vi "Ribbon Control.vi"() -> ()   [LabVIEW 2014]
panel:
  in  "1":bool
  in  "0":bool
  out "Tab Control":enum32{"0", "1"}(tab)
  in  "Tab 1 Group 2":enum32{"Page 2"}(tab)
  in  "Button Rack Center 4":bool
  in  "Button Rack Center 3":bool
  in  "Button Rack Right 2":bool
  in  "Button Rack Left 2":bool
  in  "Button Rack Center 2":bool
  in  "Button Rack Right":bool
  in  "Button Rack Left":bool
  in  "Button Rack Center":bool
  in  "String":string
  out "Ring 2":u16(ring)
  in  "Tab 1 Group 1":enum32{"Page 2"}(tab)
  in  "Add Button":bool
  in  "Save Button":bool
  in  "New Button":bool
  out "Ring":u16(ring)
  in  "Tab 2 Group 1":enum32{"Page 2"}(tab)
  in  "Add Button 3":bool
  in  "Save Button 3":bool
  in  "New Button 3":bool
  in  "Add Button 2":bool
  in  "Save Button 2":bool
  in  "New Button 2":bool
  out "Ring 3":u16(ring)
  out "Waveform Graph":dynamicdata(graph)
  in  "Frequency":dbl(slide) scale=0.0..10.0 scale format="%#_6p"
  in  "Amplitude":dbl(slide) scale=0.0..10.0
  in  "stop":bool
  # "Tab 1"
  # "Group Title"
  # "Group Title"
  # "Tab 2"
  # "Group Title"
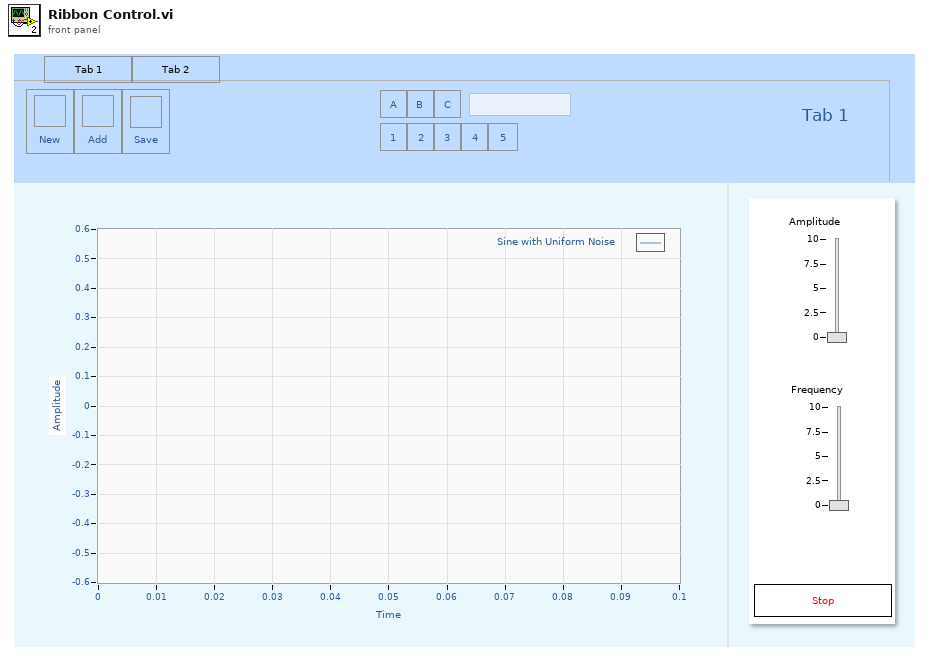
[diagram p1: front panel]
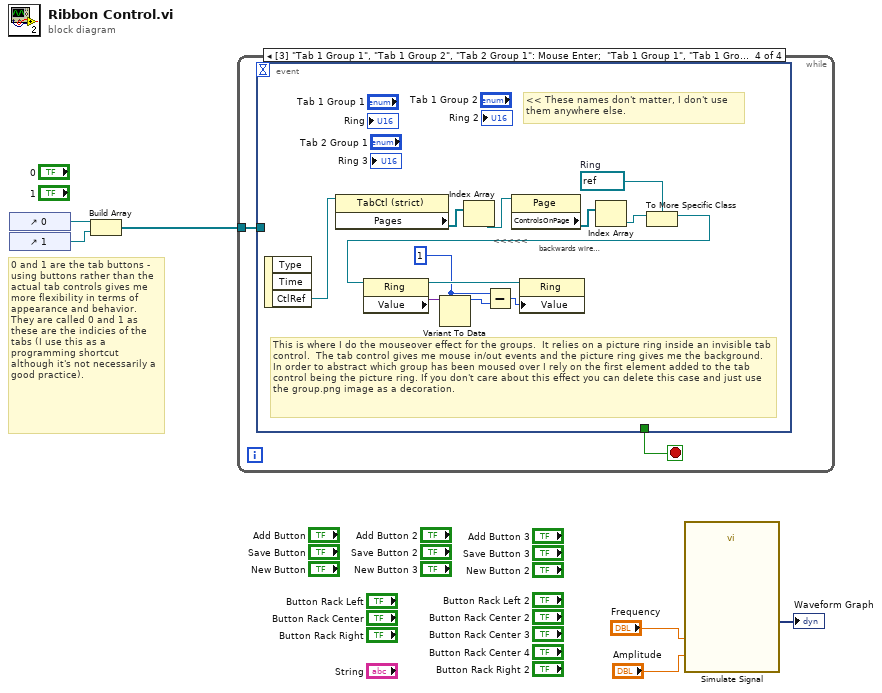
[diagram p0: block diagram]
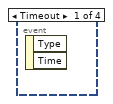
[diagram p2: hidden frame]
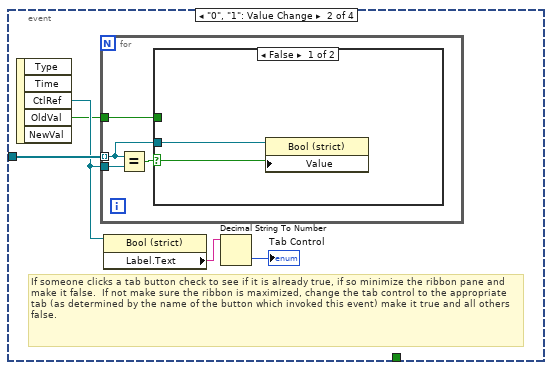
[diagram p3: hidden frame]
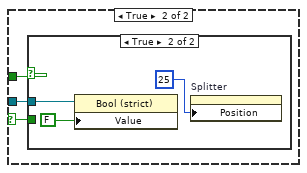
[diagram p4: hidden frame]
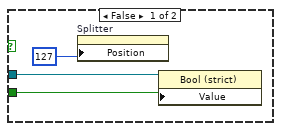
[diagram p5: hidden frame]
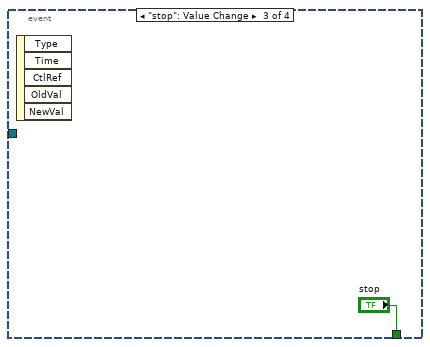
[diagram p6: hidden frame]
diagram:
  # "0 and 1 are the tab buttons - using buttons rather than the actual tab controls gives me more flexibility in terms of appearance and behavior.  They are called 0 and 1 as these are the indicies of the tabs (I use this as a programming shortcut although it's not necessarily a good practice)."
  n1 = control-ref of="0"() -> (w6:refnum<vi>)
  n2 = control-ref of="1"() -> (w5:refnum<vi>)
  n3 = Build Array(w6, w5) -> (w4:refnum<vi>[])
  n4 = while {
    tunnel: w4 -> [w8]
    stop <- w7 stop-if-true
    n5 = event shown="[3] \"Tab 1 Group 1\", \"Tab 1 Group 2\", \"Tab 2 Group 1\": Mouse Enter;  \"Tab 1 Group 1\", \"Tab 1 Group 2\", \"Tab 2 Group 1\": Mouse Leave" {
      selector: _ -> [_ _ _ _]
      dyn-events: _ -> [_ _ _ _]
      timeout: _ -> [_ _ _ _]
      tunnel: w8 -> [_ w11 _ _]
      tunnel: [_ _ "stop" _] -> w7
      event Timeout {
        n6 = event-data() -> ()  [unwired: 1 in, 2 out]
      }
      event "0", "1": Value Change {
        # "If someone clicks a tab button check to see if it is already true, if so minimize the ribbon pane and make it false.  If not make sure the ribbon is maximized, change the tab control to the appropriate tab (as determined by the name of the button which invoked this event) make it true and all others false."
        n7 = event-data() -> ("CtlRef"=w10:refnum<vi>, "OldVal"=w9:bool)  [unwired: 1 in, 3 out]
        n8 = for {
          tunnel: w11 -> [w16] mode=indexing
          tunnel: w10 -> [w17]
          tunnel: w9 -> [w14]
          n9 = Equal?(x=w16, y=w17) -> (x = y?=w15:bool)
          n10 = case shown="False" w15 {
            selector: w15 -> [w18 w22]
            tunnel: w16 -> [w19 w21]
            tunnel: w14 -> [_ w20]
            frame False {
              n11 = property on="Property Node" class="Bool (strict)"(reference=w19, "Value"=w18) -> ()  [unwired: 1 in, 2 out]
            }
            frame True {
              n12 = case shown="True" w20 {
                tunnel: w22 -> [w25 _]
                tunnel: w21 -> [w24 w27]
                frame False {
                  n13 = property on="Splitter" class="Splitter"("Position"=127 ("Splitter Position")) -> ()  [unwired: 2 in, 2 out]
                  n14 = property on="Property Node" class="Bool (strict)"(reference=w24, "Value"=w25) -> ()  [unwired: 1 in, 2 out]
                }
                frame True {
                  n15 = property on="Property Node" class="Bool (strict)"(reference=w27, "Value"=FALSE) -> ()  [unwired: 1 in, 2 out]
                  n16 = property on="Splitter" class="Splitter"("Position"=25 ("Splitter Position")) -> ()  [unwired: 2 in, 2 out]
                }
              }
            }
          }
        }
        n17 = property class="Bool (strict)"(reference=w10) -> ("Label.Text"=w13:string)  [unwired: 1 in, 2 out]
        n18 = Decimal String To Number(string=w13) -> (number=→"Tab Control":i32)  [unwired: 2 in, 1 out]
      }
      event "stop": Value Change {
        n19 = event-data() -> ()  [unwired: 1 in, 5 out]
      }
      event "Tab 1 Group 1", "Tab 1 Group 2", "Tab 2 Group 1": Mouse Enter; "Tab 1 Group 1", "Tab 1 Group 2", "Tab 2 Group 1": Mouse Leave {
        w31 = u16 1 ("Ring")
        w36 = refnum<vi> refnum  # Ring
        # "backwards wire (sorry!)"
        # "<< These names don't matter, I don't use\nthem anywhere else."
        # "This is where I do the mouseover effect for the groups.  It relies on a picture ring inside an invisible tab control.  The tab control gives me mouse in/out events and the picture ring gives me the background.  In order to abstract which group has been moused over I rely on the first element added to the tab control being the picture ring. If you don't care about this effect you can delete this case and just use the group.png image as a decoration."
        # "<<<<<"
        n20 = event-data() -> ("CtlRef"=w41:refnum<vi>)  [unwired: 1 in, 2 out]
        n21 = property class="TabCtl (strict)"(reference=w41) -> ("Pages"=w40:refnum<vi>[])  [unwired: 1 in, 2 out]
        n22 = Index Array(array=w40) -> (element=w39:refnum<vi>)  [unwired: 1 in]
        n23 = property class="Page"(reference=w39) -> ("ControlsOnPage"=w38:refnum<vi>[])  [unwired: 1 in, 2 out]
        n24 = Index Array(array=w38) -> (element=w37:refnum<vi>)  [unwired: 1 in]
        n25 = To More Specific Class(target class=w36, reference=w37) -> (specific class reference=w35:refnum<vi>)  [unwired: 1 in, 1 out]
        n26 = property class="Ring"(reference=w35) -> (reference out=w34:refnum<vi>, "Value"=w32:variant)  [unwired: 1 in, 1 out]
        n27 = Variant To Data(type=w31, Variant=w32) -> (data=w30:u16)  [unwired: 1 in, 1 out]
        n28 = Subtract(x=w31, y=w30) -> (x-y=w33:u16)
        n29 = property class="Ring"(reference=w34, "Value"=w33) -> ()  [unwired: 1 in, 2 out]
      }
    }
  }
  n30 = call "Simulate Signal"("Frequency"="Frequency", "Amplitude"="Amplitude") -> ("Sine with Uniform Noise"=→"Waveform Graph":dynamicdata)  [unwired: 12 in, 1 out]
